vi "Init.vi"(10 "Input":T4) -> (2 "Msg":T1 {"Teller"."Absolute Time" format="%<%x %.3X>T"})   [LabVIEW 2020, in "_Template.lvlib" / "Templates.lvlib" / "TEMPLATE jettl Msg.lvlib"]
uses:
  TEMPLATE jettl Msg.lvlib
  jettl/jettl/Msg/Msg.lvclass
  jettl/jettl/Msg Input/Msg Input.lvclass
  jettl/jettl/Msg Output/Msg Output.lvclass
  TEMPLATE Msg Output/TEMPLATE Msg Output.lvclass
  TEMPLATE Msg/TEMPLATE Msg.lvclass
  TEMPLATE Msg Input/TEMPLATE Msg Input.lvclass
  jettl/jettl/Unified Actor Relation.ctl
  jettl/jettl/jettl.lvlib
  jettl/jettl/Teller.ctl
  jettl/jettl/Msg.ctl
  Input.ctl
panel:
  # "This front panel should not be manipulated."
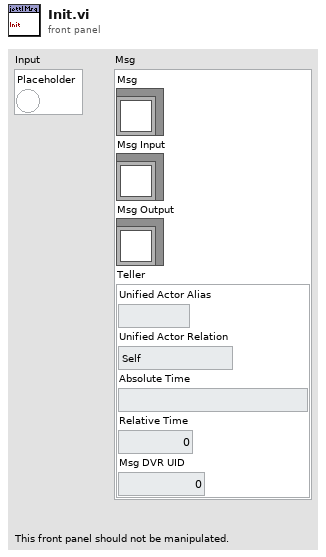
[diagram p1: front panel]
types:
  T1 = typedef "jettl.lvlib/Msg.ctl" = cluster{"Msg":refnum<class "Msg.lvclass">, "Msg Input":refnum<class "Msg Input.lvclass">, "Msg Output":refnum<class "Msg Output.lvclass">, "Teller":T2}
  T2 = typedef "jettl.lvlib/Teller.ctl" = cluster{"Unified Actor Alias":string, "Unified Actor Relation":T3, "Absolute Time":timestamp, "Relative Time":dbl, "Msg DVR UID":i32}
  T3 = typedef "jettl.lvlib/Unified Actor Relation.ctl" = enum16{"Self", "Parent", "Child"}
  T4 = typedef "_Template.lvlib/Templates.lvlib/TEMPLATE jettl Msg.lvlib/Input.ctl" = cluster{"Placeholder":bool}
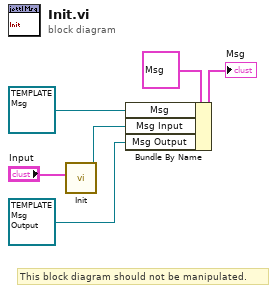
[diagram p0: block diagram]
diagram:
  # "This block diagram should not be manipulated."
  n1 = call "Init.vi"("Input"="Input") -> ("TEMPLATE Msg Input out"=w2:refnum<class "TEMPLATE Msg Input.lvclass">)  [unwired: 10 in]
  n2 = Bundle By Name(cluster=T1 {"Msg"=refnum, "Msg Input"=refnum, "Msg Output"=refnum, "Teller"={"Unified Actor Alias"="", "Unified Actor Relation"=enum."Self", "Absolute Time"=timestamp(0 s since 1904-01-01), "Relative Time"=0.0, "Msg DVR UID"=0}} ("Msg Attributes"), "Msg"=refnum<class "TEMPLATE Msg.lvclass"> refnum ("_Template.lvlib:Templates.lvlib:TEMPLATE jettl Msg.lvlib:TEMPLATE Msg.lvlib:TEMPLATE Msg.lvclass"), "Msg Input"=w2, "Msg Output"=refnum<class "TEMPLATE Msg Output.lvclass"> refnum ("_Template.lvlib:Templates.lvlib:TEMPLATE jettl Msg.lvlib:TEMPLATE Msg Output.lvclass")) -> (→"Msg":T1)
